vi "Lc_2024.vi"(3 "d^2Cw(T)/dT^2":dbl, 4 "d^2Cd(T)/dT^2":dbl, 5 "dCw(T)/dT":dbl, 6 "dCd(T)/dT":dbl, 7 "Cw(T)":dbl, 8 "Cd(T)":dbl, 9 "Gamma0_water":dbl, 10 "Gamma0_dry air":dbl, 11 "Temperature [K]":dbl) -> (0 "Lcw":dbl, 2 "Lcd":dbl)   [LabVIEW 2016]
uses:
  SOS_Global_2022.vi
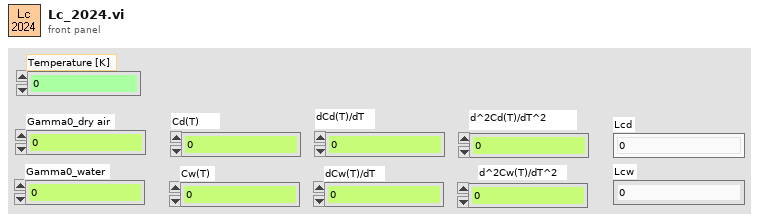
[diagram p1: front panel]
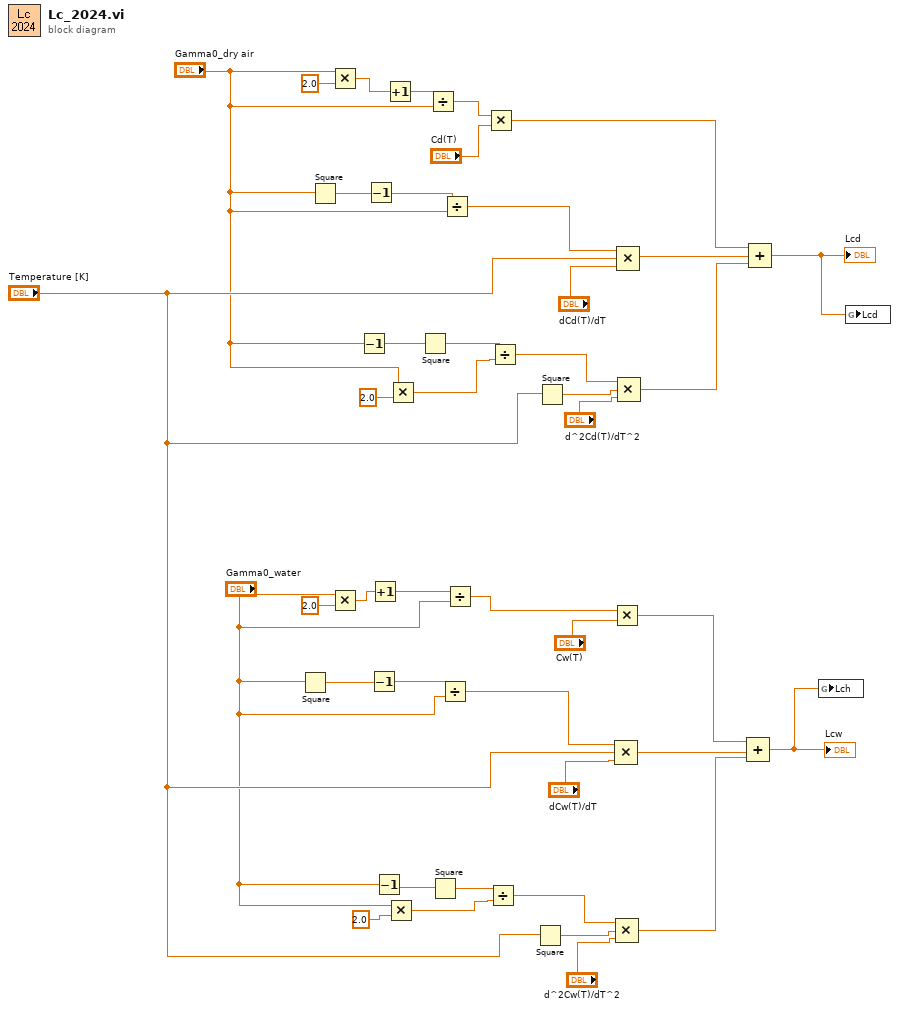
[diagram p0: block diagram]
diagram:
  n1 = Square(x="Gamma0_water") -> (x^2=w4:dbl)
  n2 = Square(x="Gamma0_dry air") -> (x^2=w10:dbl)
  n3 = Multiply(x="Gamma0_dry air", y=2.0) -> (x*y=w12:dbl)
  n4 = Multiply(x="Gamma0_water", y=2.0) -> (x*y=w6:dbl)
  n5 = Decrement(x="Gamma0_dry air") -> (x-1=w7:dbl)
  n6 = Decrement(x=w10) -> (x-1=w9:dbl)
  n7 = Decrement(x=w4) -> (x-1=w3:dbl)
  n8 = Increment(x=w6) -> (x+1=w5:dbl)
  n9 = Decrement(x="Gamma0_water") -> (x-1=w1:dbl)
  n10 = Increment(x=w12) -> (x+1=w11:dbl)
  n11 = Multiply(x="Gamma0_water", y=2.0) -> (x*y=w24:dbl)
  n12 = Multiply(x="Gamma0_dry air", y=2.0) -> (x*y=w36:dbl)
  n13 = Square(x=w7) -> (x^2=w38:dbl)
  n14 = Divide(x=w11, y="Gamma0_dry air") -> (x/y=w42:dbl)
  n15 = Square(x=w1) -> (x^2=w26:dbl)
  n16 = Divide(x=w3, y="Gamma0_water") -> (x/y=w27:dbl)
  n17 = Divide(x=w9, y="Gamma0_dry air") -> (x/y=w40:dbl)
  n18 = Divide(x=w5, y="Gamma0_water") -> (x/y=w28:dbl)
  n19 = Multiply(x=w42, y="Cd(T)") -> (x*y=w32:dbl)
  n20 = Divide(x=w26, y=w24) -> (x/y=w23:dbl)
  n21 = Divide(x=w38, y=w36) -> (x/y=w35:dbl)
  n22 = Square(x="Temperature [K]") -> (x^2=w22:dbl)
  n23 = Square(x="Temperature [K]") -> (x^2=w34:dbl)
  n24 = Multiply(x=w28, y="Cw(T)") -> (x*y=w21:dbl)
  n25 = Compound Arithmetic op=MULTIPLY(w27, "Temperature [K]", "dCw(T)/dT") -> (w20:dbl)
  n26 = Compound Arithmetic op=MULTIPLY(w23, w22, "d^2Cw(T)/dT^2") -> (w19:dbl)
  n27 = Compound Arithmetic op=MULTIPLY(w40, "Temperature [K]", "dCd(T)/dT") -> (w31:dbl)
  n28 = Compound Arithmetic op=MULTIPLY(w35, w34, "d^2Cd(T)/dT^2") -> (w30:dbl)
  n29 = Compound Arithmetic op=ADD(w21, w20, w19) -> (w13:dbl)
  "Lcw" <- w13
  n30 = Compound Arithmetic op=ADD(w32, w31, w30) -> (w14:dbl)
  "Lcd" <- w14
  n31 = global write "SOS_Global_2022.vi" "Lch"(w13) -> ()
  n32 = global write "SOS_Global_2022.vi" "Lcd"(w14) -> ()
